vi "GVUTC.vi"() -> ()   [LabVIEW 2017]
panel:
  out "GV UTC":dbl
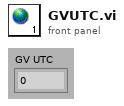
[diagram p1: front panel]
diagram:
